vi "SOC_calculator (SubVI).vi"(1 "Capacity Usable":dbl=10.0, 2 "SOC init":dbl, 3 "Current":dbl=600.0) -> (0 "Waveform Graph":dbl[](graph))   [LabVIEW 2017]
uses:
  <vilib>/Analysis/NI_AALPro.lvlib
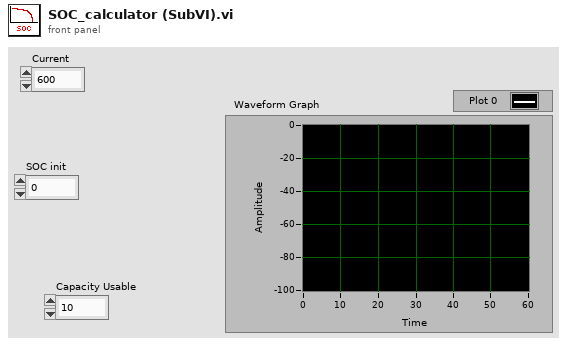
[diagram p1: front panel]
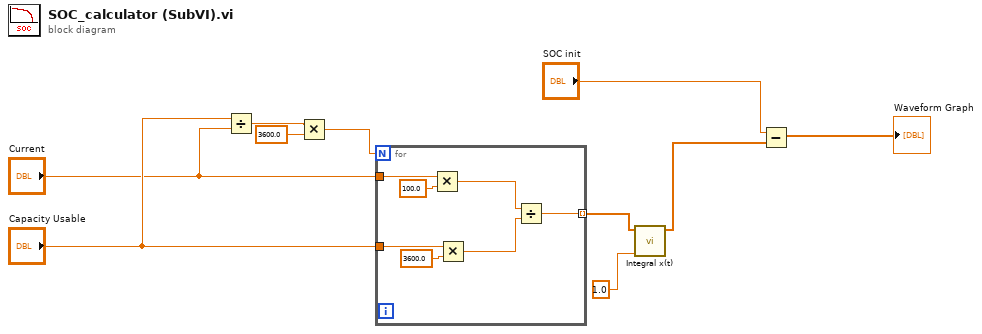
[diagram p0: block diagram]
diagram:
  n1 = Divide(x="Capacity Usable", y="Current") -> (x/y=w3:dbl)
  n2 = Multiply(x=w3, y=3600.0) -> (x*y=w2:dbl)
  n3 = for {
    N: w2 -> [_]
    tunnel: "Capacity Usable" -> [w17]
    tunnel: "Current" -> [w15]
    tunnel: [w11] -> w10 mode=indexing
    n4 = Multiply(x=w15, y=100.0) -> (x*y=w13:dbl)
    n5 = Multiply(x=w17, y=3600.0) -> (x*y=w12:dbl)
    n6 = Divide(x=w13, y=w12) -> (x/y=w11:dbl)
  }
  n7 = call <vilib>:"Integral x(t).vi"("dt"=1.0, "X"=w10) -> ("Integral X"=w8:dbl[])  [unwired: 8 in, 1 out]
  n8 = Subtract(x="SOC init", y=w8) -> (x-y=→"Waveform Graph":dbl[])
